vi "Get VI Qualified Name.vi"(8 "错误输入（无错误）":errorcluster, 11 "VI Path":path) -> (0 "错误输出":errorcluster, 3 "VI Qualified Name":string)   [LabVIEW 2012, in "Application.lvlib"]
uses:
  Application.lvlib
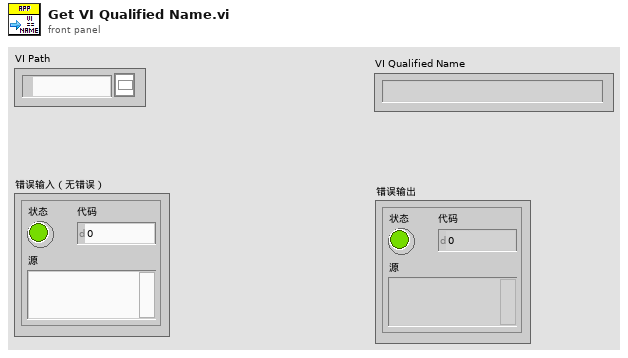
[diagram p1: front panel]
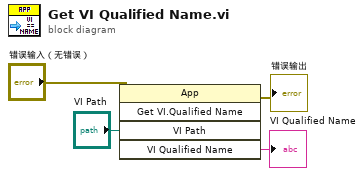
[diagram p0: block diagram]
diagram:
  n1 = invoke class="App" method="Get VI.Qualified Name"(error in="错误输入（无错误）", "VI Path"="VI Path") -> (error out=→"错误输出":errorcluster, "VI Qualified Name"=→"VI Qualified Name":string)  [unwired: 3 in, 3 out]
